vi "Example TCP Client-Server.vi"() -> ()   [LabVIEW 2013]
uses:
  <vilib>/LabVIEW Open Source Project/MQTT Connection/MQTT_Connection/Connection/Connection.lvclass
  MQTT_TCP/Connection/TCPConnection.lvclass
panel:
  out "server connected":bool
  out "client connected":bool
  out "Comm OK":bool
  out "value":dbl
  out "listener error":errorcluster
  out "client session error":errorcluster
  out "server session error":errorcluster
  out "Bytes":u8[](array[numeric]) format="%08b"
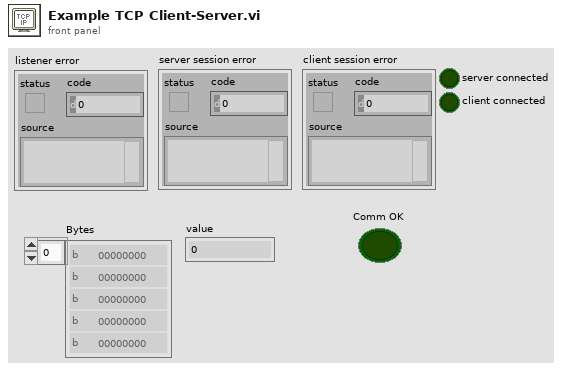
[diagram p1: front panel]
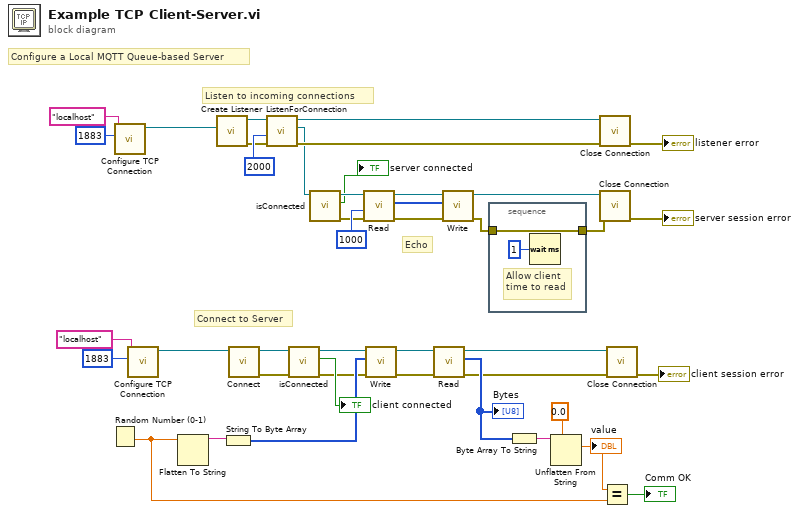
[diagram p0: block diagram]
diagram:
  # "Connect to Server"
  # "Echo"
  # "Listen to incoming connections"
  # "Configure a Local MQTT Queue-based Server"
  n1 = Random Number (0-1)() -> (number: 0 to 1=w13:dbl)
  n2 = call "Configure TCP Connection.vi"("remote port (80)"=u16 1883, "address (localhost)"="localhost") -> ("TCPConnection"=w20:refnum<class "TCPConnection.lvclass">)  [unwired: 8 in, 1 out]
  n3 = call "Configure TCP Connection.vi"("remote port (80)"=u16 1883, "address (localhost)"="localhost") -> ("TCPConnection"=w19:refnum<class "TCPConnection.lvclass">)  [unwired: 8 in, 1 out]
  n4 = Flatten To String(anything=w13) -> (data string=w30:string)  [unwired: 3 in, 2 out]
  n5 = call <vilib>:"Create Listener.vi"("Connection Configuration"=w20) -> ("error out"=w39:errorcluster, "Listener"=w42:refnum<class "Connection.lvclass">)  [unwired: 9 in]
  n6 = String To Byte Array(string=w30) -> (unsigned byte array=w29:u8[])
  n7 = call <vilib>:"Connect.vi"("Connection in"=w19) -> ("error out"=w8:errorcluster, "Connection out"=w6:refnum<class "TCPConnection.lvclass">)  [unwired: 9 in]
  n8 = call <vilib>:"ListenForConnection.vi"("error in (no error)"=w39, "timeout (2000 ms)"=2000 ("bytes to read (100)"), "Listener"=w42) -> ("error out"=w24:errorcluster, "Connection"=w4:refnum<class "Connection.lvclass">, "Listener out"=w40:refnum<class "Connection.lvclass">)  [unwired: 5 in, 1 out]
  n9 = call <vilib>:"isConnected.vi"("error in (no error)"=w8, "Connection in"=w6) -> ("error out"=w7:errorcluster, "connected"=→"client connected":bool, "Connection out"=w5:refnum<class "TCPConnection.lvclass">)  [unwired: 7 in]
  n10 = call <vilib>:"isConnected.vi"("Connection in"=w4) -> ("error out"=w2:errorcluster, "connected"=→"server connected":bool, "Connection out"=w3:refnum<class "Connection.lvclass">)  [unwired: 8 in]
  n11 = call <vilib>:"Read.vi"("error in (no error)"=w2, "timeout (5000 ms)"=1000 ("bytes to read (100)"), "TCPConnection in"=w3) -> ("error out"=w34:errorcluster, "Bytes"=w36:u8[], "TCPConnection out"=w37:refnum<class "Connection.lvclass">)  [unwired: 4 in, 2 out]
  n12 = call <vilib>:"Write.vi"("error in (no error)"=w7, "Bytes"=w29, "Connection in"=w5) -> ("error out"=w33:errorcluster, "Connection"=w35:refnum<class "TCPConnection.lvclass">)  [unwired: 7 in]
  n13 = call <vilib>:"Read.vi"("error in (no error)"=w33, "TCPConnection in"=w35) -> ("error out"=w22:errorcluster, "Bytes"=w28:u8[], "TCPConnection out"=w21:refnum<class "TCPConnection.lvclass">)  [unwired: 5 in, 2 out]
  "Bytes" <- w28
  n14 = call <vilib>:"Write.vi"("error in (no error)"=w34, "Bytes"=w36, "Connection in"=w37) -> ("error out"=w11:errorcluster, "Connection"=w31:refnum<class "Connection.lvclass">)  [unwired: 7 in]
  n15 = stacked-sequence {
    tunnel: w11 -> [w43]
    tunnel: [w43] -> w10
    frame #0 {
      # "Allow client\ntime to read"
      n16 = Wait (ms)(milliseconds to wait=u32 1) -> ()  [unwired: 1 out]
    }
  }
  n17 = Byte Array To String(unsigned byte array=w28) -> (string=w27:string)
  n18 = Unflatten From String(type=0.0, binary string=w27) -> (value=w14:dbl)  [unwired: 3 in, 2 out]
  "value" <- w14
  n19 = call <vilib>:"Close Connection.vi"("error in (no error)"=w24, "Connection in"=w40) -> ("error out"=→"listener error":errorcluster)  [unwired: 8 in, 1 out]
  n20 = call <vilib>:"Close Connection.vi"("error in (no error)"=w10, "Connection in"=w31) -> ("error out"=→"server session error":errorcluster)  [unwired: 8 in, 1 out]
  n21 = Equal?(x=w14, y=w13) -> (x = y?=→"Comm OK":bool)
  n22 = call <vilib>:"Close Connection.vi"("error in (no error)"=w22, "Connection in"=w21) -> ("error out"=→"client session error":errorcluster)  [unwired: 8 in, 1 out]
